vi "AMWaveFINAL.vi"(10 "Digitizing Parameters":T2) -> (2 "AM Wave":cluster{"Time":dbl[], "Displacement":dbl[]} {"Displacement" format="%#_3g"; "Time" format="%#.3g"})   [LabVIEW 2014]
doc: "Plots an N element array of displacement values for an amplitude-modulated (AM) wave. \n\nTypical AM wave has signal frequency >> modulation frequency."
uses:
  <vilib>/imath/engines/lvmath2/RunTimeEngine/Managers/WorkSpace/UID Generator.vi
  <vilib>/imath/engines/lvmath2/RunTimeEngine/RunTimeType/NIMS_RunTimeType_From StrictType (excl LVString).vi
  <instcachedir>/0/NIMS_RunTimeType_From StrictType (excl LVString)_6F30FCEAD152B34FB6BC3D48AAFE00E6.lvgen/NIMS_RunTimeType_From StrictType (excl LVString)_6F30FCEAD152B34FB6BC3D48AAFE00E6_000.vi
  <vilib>/imath/engines/lvmath2/RunTimeEngine/LocalVariableDefStatement/MC_LocalVariableDefStatement_Display.vi
  <vilib>/imath/engines/lvmath2/RunTimeEngine/RangeToken/NIMS_Range.vi
  <instcachedir>/0/NIMS_Range_6DDDFF7386AB584A9063FA25EAF603C1.lvgen/NIMS_Range_6DDDFF7386AB584A9063FA25EAF603C1_000.vi
  <vilib>/imathl/engines/lvmath/Functions/Error Handling/Create Error.vi
  <vilib>/imath/engines/lvmath2/RunTimeEngine/ArithmeticOperatorToken/NIMS_ArithmeticOperator_times.vi
  <instcachedir>/0/NIMS_ArithmeticOperator_times_831F30C6BFCCF94698B6F46369084E97.lvgen/NIMS_ArithmeticOperator_times_831F30C6BFCCF94698B6F46369084E97_000.vi
  <vilib>/imath/engines/lvmath2/RunTimeEngine/Managers/SymbolTable/Clear UID.vi
  <vilib>/imath/engines/lvmath2/RunTimeEngine/NodeEndStatement/NIMS_NodeEndStatement_Output.vi
  <instcachedir>/0/NIMS_NodeEndStatement_Output_53EC0D466D134D7ABD903AC30B43404B.lvgen/NIMS_NodeEndStatement_Output_53EC0D466D134D7ABD903AC30B43404B_005.vi
  <vilib>/imath/engines/lvmath2/RunTimeEngine/ErrorHandling/NIMS_Finalize Error.vi
  <vilib>/imath/engines/lvmath2/RunTimeEngine/Managers/SymbolTable/NIMS_WorkSpace.lvlib
panel:
  in  "AM Wave Parameters":T1
  out "XY Graph":cluster{"t":dbl[], "x":dbl[]}(graph)
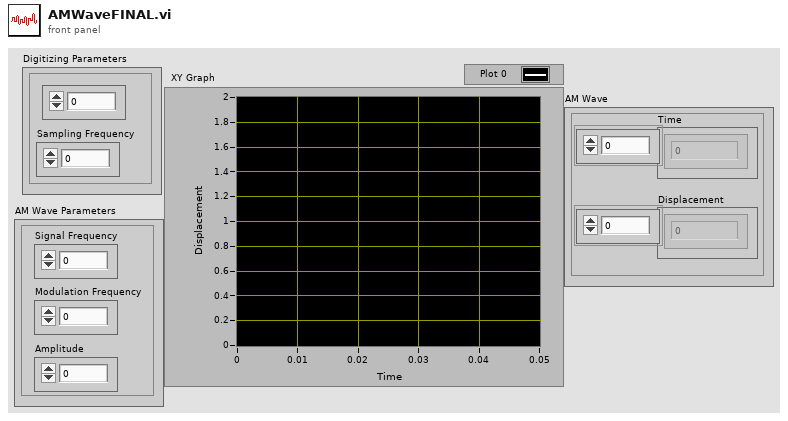
[diagram p1: front panel]
types:
  T1 = cluster{"Signal Frequency":dbl, "Modulation Frequency":dbl, "Amplitude":dbl}
  T2 = cluster{"Number of Samples":i32, "Sampling Frequency":dbl}
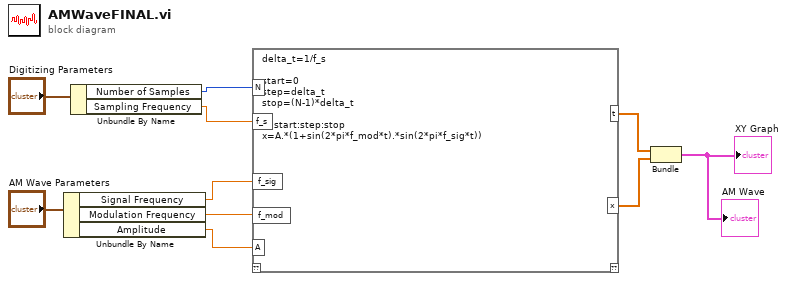
[diagram p0: block diagram]
diagram:
  n1 = Unbundle By Name("AM Wave Parameters") -> ("Signal Frequency"=w3:dbl, "Modulation Frequency"=w2:dbl, "Amplitude"=w1:dbl)
  n2 = Unbundle By Name("Digitizing Parameters") -> ("Number of Samples"=w7:i32, "Sampling Frequency"=w6:dbl)
  n3 = mathscript code="delta_t=1/f_s\n\nstart=0\nstep=delta_t\nstop=(N-1)*delta_t\n\nt=start:step:stop\nx=A.*(1+sin(2*pi*f_mod*t).*sin(2*pi*f_sig*t))"("N"=w7, "f_s"=w6, "f_sig"=w3, "f_mod"=w2, "A"=w1) -> ("t"=w10:dbl[], "x"=w9:dbl[])  [unwired: 1 in, 1 out]
  n4 = Bundle("t"=w10, "x"=w9) -> (→"XY Graph" →"AM Wave":cluster{"t":dbl[], "x":dbl[]})  [unwired: 1 in]
